vi "Erase Message.vi"(8 "error in (no error)":errorcluster, 11 "SPARC4_GUI in":refnum<class "S4GEI.lvclass">) -> (0 "error out":errorcluster, 3 "SPARC4_GUI out":refnum<class "S4GEI.lvclass">)   [LabVIEW 2018, in "S4GEI.lvclass"]
uses:
  S4GEI.lvclass
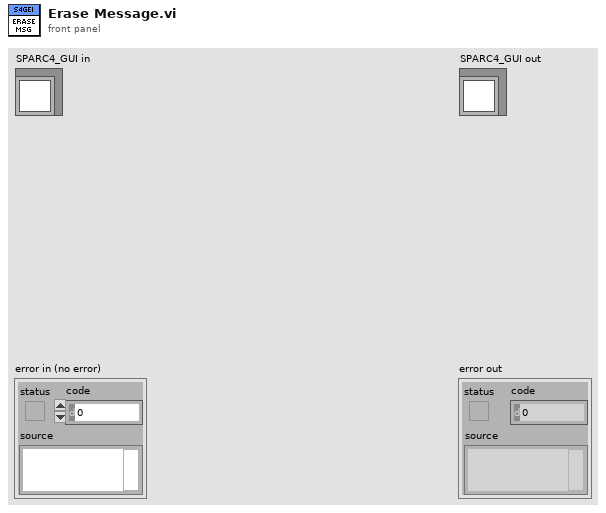
[diagram p1: front panel]
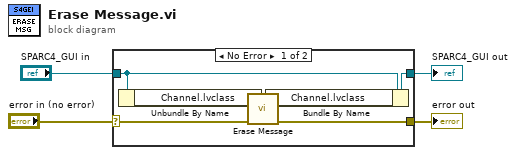
[diagram p0: block diagram]
diagram:
  n1 = case shown="No Error" "error in (no error)" {
    selector: "error in (no error)" -> [w5 w12]
    tunnel: [w6 w12] -> w3
    tunnel: [w9 w11] -> w1
    tunnel: "SPARC4_GUI in" -> [w10 w11]
    frame No Error {
      n2 = Unbundle By Name(w10) -> ("Channel.lvclass"=w8:refnum<class "Channel.lvclass">)
      n3 = call "Erase Message.vi"("error in (no error)"=w5, "Channel GUI in"=w8) -> ("error out"=w6:errorcluster, "Channel GUI out"=w7:refnum<class "Channel.lvclass">)  [unwired: 8 in]
      n4 = Bundle By Name(cluster=w10, "Channel.lvclass"=w7) -> (w9:refnum<class "S4GEI.lvclass">)
    }
    frame Error {
    }
  }
  "error out" <- w3
  "SPARC4_GUI out" <- w1
